vi "Launcher.vi"   [LabVIEW 2017]
types:
  T1 = enum32{"Invalid", "Standard", "Closed", "Hidden", "Minimized", "Maximized"}
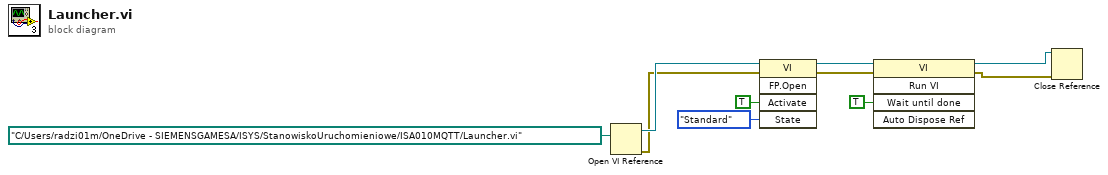
[diagram p0: block diagram]
diagram:
  n1 = Open VI Reference(vi path=path "C:/Users/radzi01m/OneDrive - SIEMENSGAMESA/ISYS/StanowiskoUruchomieniowe/ISA010MQTT/Launcher.vi") -> (vi reference=w9:refnum<vi>, error out=w3:errorcluster)  [unwired: 5 in]
  n2 = invoke class="VI" method="FP.Open"(reference=w9, error in=w3, "Activate"=TRUE ("Activate?"), "State"=T1."Standard") -> (reference out=w8:refnum<vi>, error out=w2:errorcluster)  [unwired: 1 in, 3 out]
  n3 = invoke class="VI" method="Run VI"(reference=w8, error in=w2, "Wait until done"=TRUE ("Wait Until Done")) -> (reference out=w6:refnum<vi>, error out=w1:errorcluster)  [unwired: 2 in, 3 out]
  n4 = Close Reference(reference=w6, error in (no error)=w1) -> ()  [unwired: 1 out]
